vi "1radar.vi"(7 "date/time string":string, 8 "Q":dbl[](array[numeric]), 10 "radar number":i32, 11 "input cluster":T1) -> (0 "error out":errorcluster, 1 "Q out":dbl[](array[numeric]), 3 "VISA resource out":refnum<visa-resource-name>, 4 "Spectrum":waveform(dbl)(graph), 5 "I/Q channels":waveform(dbl)(graph))   [LabVIEW 2015]
uses:
  <vilib>/Analysis/2dsp.llb/Real FFT.vi
  <vilib>/measure/madcrms.llb/Basic Averaged DC-RMS for 1 Chan.vi
  <vilib>/measure/NI_MAPro.lvlib
  <vilib>/Analysis/NI_AALPro.lvlib
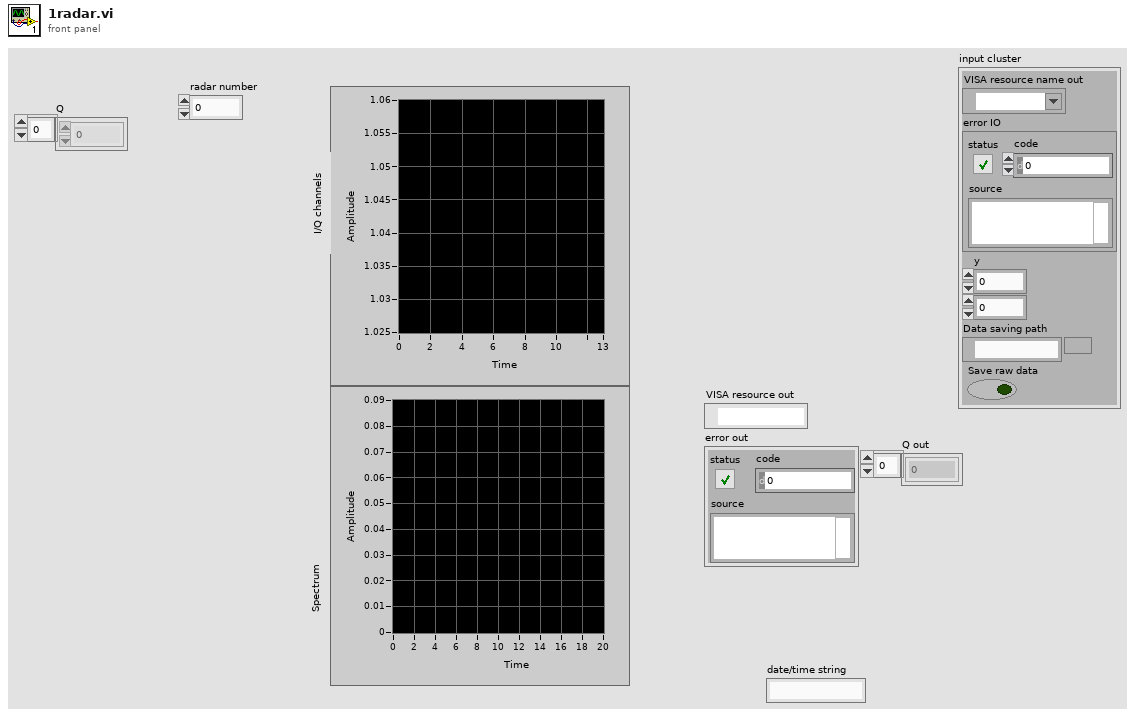
[diagram p1: front panel]
types:
  T1 = cluster{"VISA resource name out":refnum<visa-resource-name>, "error IO":errorcluster, "y":u8, i32, "Data saving path":path, "Save raw data":bool}
  T2 = enum16{"open", "replace", "create", "open or create", "replace or create", "replace or create with confirmation"}
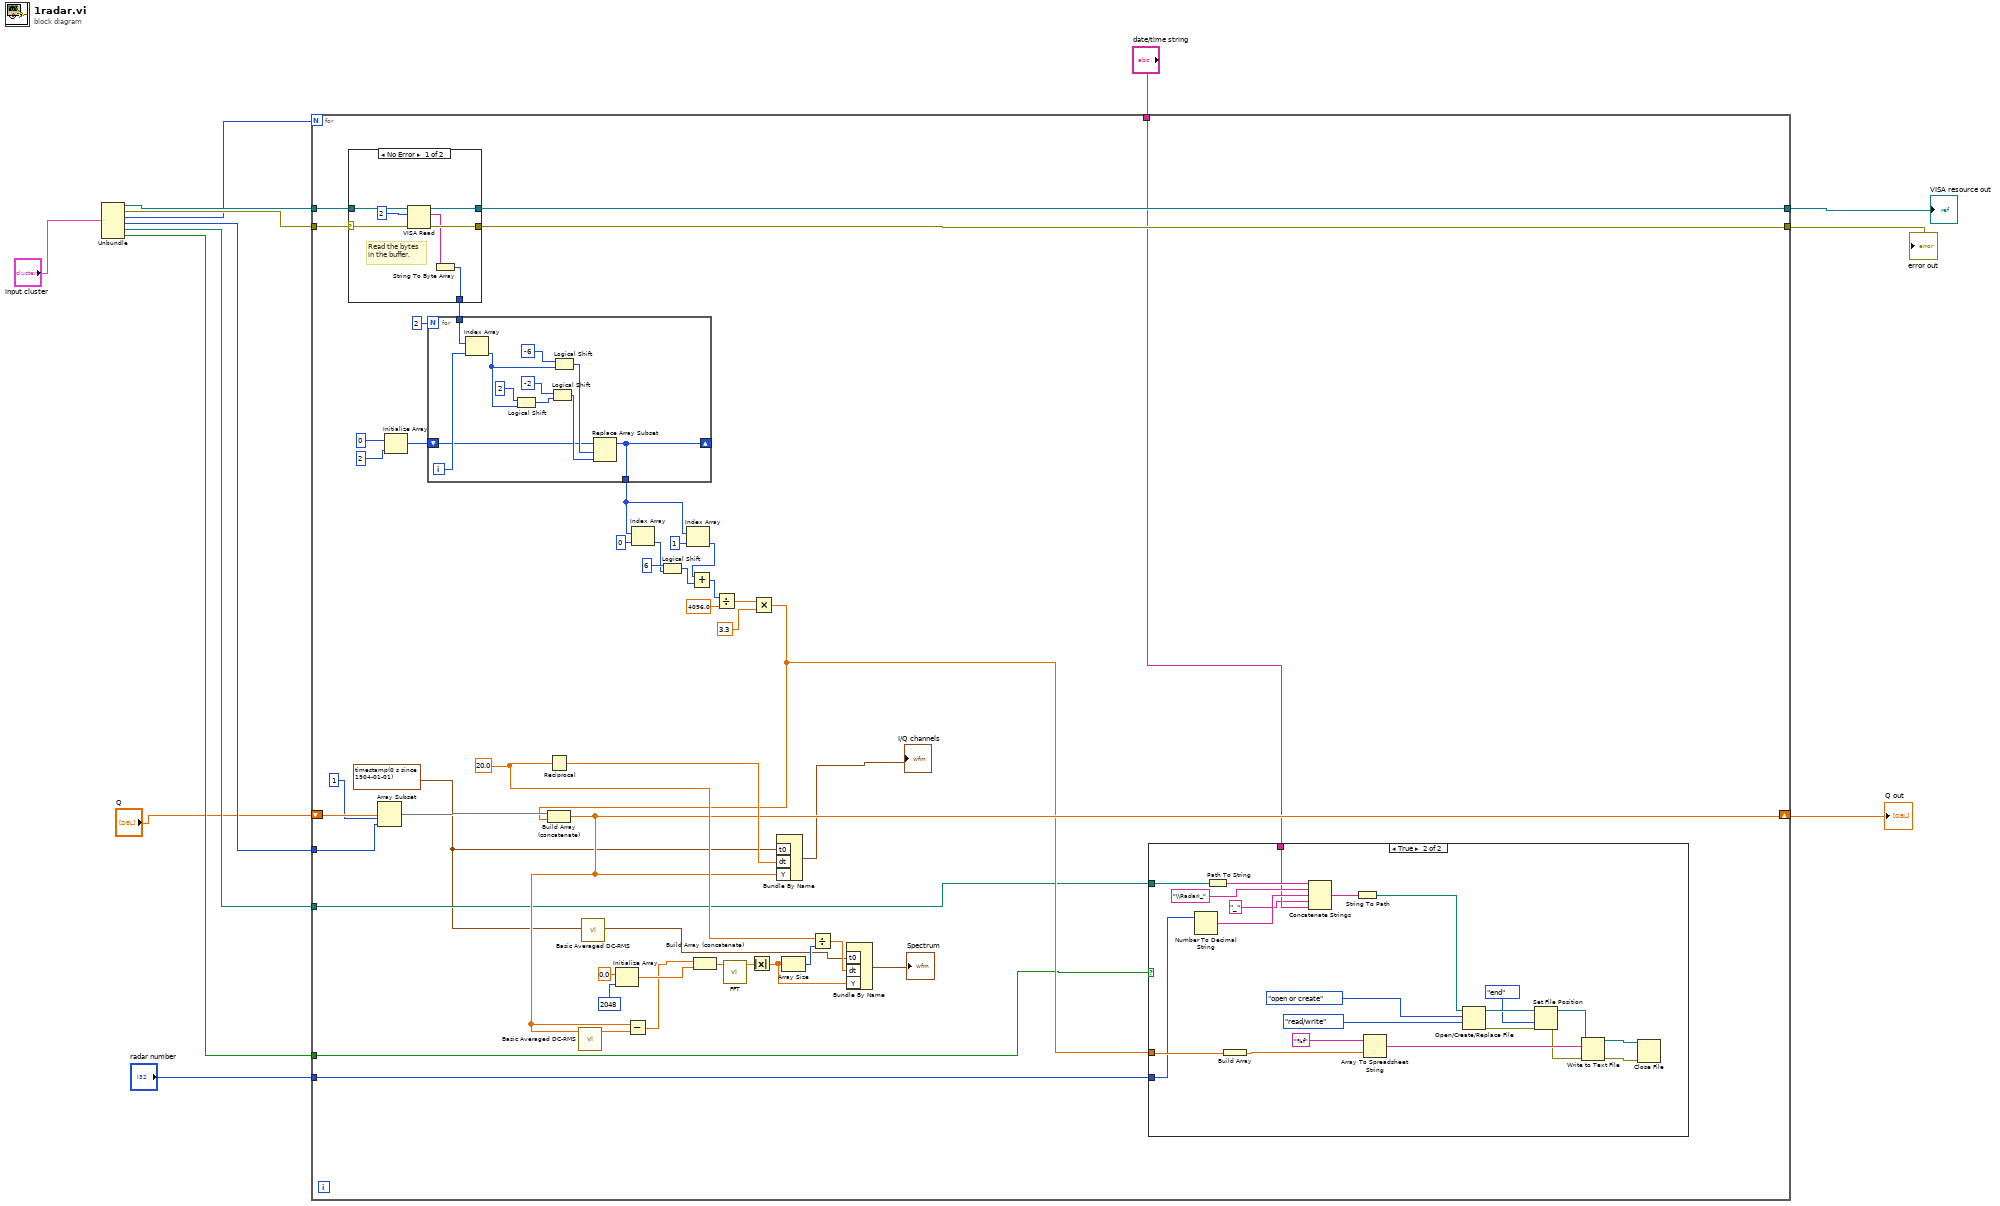
[diagram p0: block diagram]
diagram:
  n1 = Unbundle("input cluster") -> ("VISA resource name out"=w9:refnum<visa-resource-name>, "error IO"=w8:errorcluster, "y"=w5:u8, w4:i32, "Data saving path"=w3:path, "Save raw data"=w2:bool)
  n2 = for {
    N: w5 -> [_]
    tunnel: w8 -> [w44]
    tunnel: w9 -> [w43]
    tunnel: [w24] -> w12
    tunnel: [w23] -> w11
    tunnel: w4 -> [w50]
    shift-right: [w29] -> w10
    shift-left: "Q" -> [w57]
    tunnel: "date/time string" -> [w21]
    tunnel: "radar number" -> [w19]
    tunnel: w3 -> [w18]
    tunnel: w2 -> [w17]
    w16 = timestamp(0 s since 1904-01-01) ("t0")
    (unwired) 0
    w36 = 20.0 ("dt")
    n3 = case "Read bytes from port." shown="No Error" w44 {
      selector: w44 -> [w95 w100]
      tunnel: [w97 w100] -> w23
      tunnel: [w98 w101] -> w24
      tunnel: w43 -> [w96 w101]
      tunnel: [w93 u8[] [] ("unsigned byte array")] -> w25
      frame No Error {
        # "Read the bytes\nin the buffer."
        n4 = VISA Read(VISA resource name=w96, byte count=u32 2, error in (no error)=w95) -> (VISA resource name out=w98:refnum<visa-resource-name>, read buffer=w94:string, error out=w97:errorcluster)  [unwired: 1 out]
        n5 = String To Byte Array(string=w94) -> (unsigned byte array=w93:u8[])
      }
      frame Error {
        # "Error occurred \nreading Bytes at \nSerial Port"
      }
    }
    n6 = Array Subset(array=w57, index=1, length=w50) -> (w58:dbl[])
    n7 = Initialize Array(i16 0 ("element"), 2 ("dimension size")) -> (w26:i16[])
    n8 = for {
      N: 2 -> [_]
      tunnel: w25 -> [w86]
      tunnel: [w81] -> w31
      shift-right: [w81] -> _
      shift-left: w26 -> [w82]
      i -> [w85]
      n9 = Index Array(array=w86, index=w85) -> (element=w89:u8)
      n10 = Logical Shift(y=i8 2, x=w89) -> (x << y=w88:u8)
      n11 = Logical Shift(y=i8 -2, x=w88) -> (x << y=w83:u8)
      n12 = Logical Shift(y=i8 -6, x=w89) -> (x << y=w84:u8)
      n13 = Replace Array Subset(array=w82, new element=w83, index=w84) -> (w81:i16[])
    }
    n14 = Reciprocal(x=w36) -> (1/x=w45:dbl)
    n15 = call-poly <vilib>:"Basic Averaged DC-RMS.vi"() -> ()  [unwired: 5 in, 7 out]
    n16 = Initialize Array(0.0 ("element"), 2048 ("dimension size")) -> (w39:dbl[])
    n17 = Index Array(array=w31, index=0) -> (element=w53:i16)
    n18 = Logical Shift(y=i16 6, x=w53) -> (x << y=w51:i16)
    n19 = Index Array(array=w31, index=1) -> (element=w52:i16)
    n20 = Add(x=w52, y=w51) -> (x+y=w22:i16)
    n21 = Divide(x=w22, y=4096.0) -> (x/y=w48:dbl)
    n22 = Multiply(x=w48, y=3.3) -> (x*y=w20:dbl)
    n23 = Build Array (concatenate)(w58, w20) -> (w29:dbl[])
    n24 = call-poly <vilib>:"Basic Averaged DC-RMS.vi"("signal in"=w29) -> ("DC value"=w47:dbl)  [unwired: 4 in, 6 out]
    n25 = Subtract(x=w29, y=w47) -> (x-y=w14:dbl[])
    n26 = Build Array (concatenate)(w14, w39) -> (w40:dbl[])
    n27 = call-poly <vilib>:"FFT.vi"("X"=w40) -> ("FFT {X}"=w37:cdb[])  [unwired: 2 in, 8 out]
    n28 = Absolute Value(x=w37) -> (abs(x)=w35:dbl[])
    n29 = Bundle By Name ("Build Waveform")("t0"=w16, "dt"=w45, "Y"=w29) -> (→"I/Q channels":waveform(dbl))  [unwired: 1 out]
    n30 = Array Size(array=w35) -> (size(s)=w38:i32)
    n31 = Divide(x=w36, y=w38) -> (x/y=w34:dbl)
    n32 = Bundle By Name("t0"=w16, "dt"=w34, "Y"=w35) -> (→"Spectrum":waveform(dbl))  [unwired: 1 out]
    n33 = case shown="True" w17 {
      tunnel: w20 -> [_ w74]
      tunnel: w21 -> [_ w61]
      tunnel: w18 -> [_ w75]
      tunnel: w19 -> [_ w60]
      frame False {
      }
      frame True {
        n34 = Number To Decimal String(number=w60) -> (decimal integer string=w62:string)  [unwired: 1 in]
        n35 = Path To String(path=w75) -> (string=w78:string)
        n36 = Build Array(w74) -> (w63:dbl[])
        n37 = Concatenate Strings(w78, "\\RadarI_" ("string"), w62, "_" ("string"), w61) -> (w80:string)
        n38 = String To Path(string=w80) -> (path=w73:path)
        n39 = Array To Spreadsheet String(array=w63, 3:"%f" ("format string")) -> (spreadsheet string=w79:string)  [unwired: 1 in]
        n40 = Open/Create/Replace File(file path (use dialog)=w73, operation (0:open)=T2."open or create", access (0:read/write)=enum16{"read/write", "read-only", "write-only"}."read/write") -> (refnum out=w72:refnum<file>, error out=w71:errorcluster)  [unwired: 3 in, 1 out]
        n41 = Set File Position(refnum=w72, from (0:start)=enum16{"start", "end", "current"}."end", error in=w71) -> (refnum out=w70:refnum<file>, error out=w69:errorcluster)  [unwired: 1 in]
        n42 = Write to Text File(file (use dialog)=w70, text=w79, error in=w69) -> (refnum out=w67:refnum<file>, error out=w66:errorcluster)  [unwired: 1 in, 1 out]
        n43 = Close File(refnum=w67, error in=w66) -> ()  [unwired: 2 out]
      }
    }
  }
  "VISA resource out" <- w12
  "error out" <- w11
  "Q out" <- w10
